vi "CRYHeader x-y cols assign.vi"(9 "Common x-axis":bool, 10 "Column assignments":cluster{"x col":i32, "y col":i32}[](array[cluster]), 11 "Header row, empty":string[](array[string])) -> (3 "Header row out":string[](array[string]))   [LabVIEW 2013]
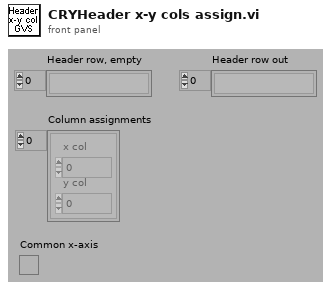
[diagram p1: front panel]
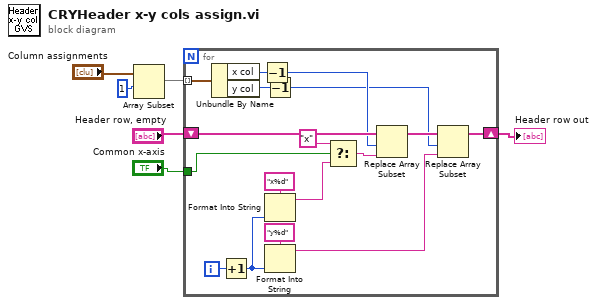
[diagram p0: block diagram]
diagram:
  n1 = Array Subset(array="Column assignments", index=1 ("Array Index")) -> (w2:cluster{"x col":i32, "y col":i32}[])  [unwired: 1 in]
  n2 = for {
    tunnel: w2 -> [w23] mode=indexing
    shift-right: [w15] -> w5
    shift-left: "Header row, empty" -> [w22]
    tunnel: "Common x-axis" -> [w10]
    i -> [w19]
    n3 = Unbundle By Name(w23) -> ("x col"=w14:i32, "y col"=w13:i32)
    n4 = Increment(x=w19) -> (x+1=w18:i32)
    n5 = Decrement(x=w14) -> (x-1=w12:i32)
    n6 = Decrement(x=w13) -> (x-1=w11:i32)
    n7 = Format Into String(format string="x%d", w18) -> (resulting string=w9:string)  [unwired: 2 in, 1 out]
    n8 = Format Into String(format string="y%d", w18) -> (resulting string=w17:string)  [unwired: 2 in, 1 out]
    n9 = Select(t="x", s=w10, f=w9) -> (s? t:f=w7:string)
    n10 = Replace Array Subset(array=w22, new element=w7, index=w12) -> (w16:string[])
    n11 = Replace Array Subset(array=w16, new element=w17, index=w11) -> (w15:string[])
  }
  "Header row out" <- w5
